vi "Set Pattern.vi"(8 "error in (no error)":errorcluster, 10 "Pattern":string, 11 "Report":refnum<class "Report.lvclass">) -> (0 "error out":errorcluster, 3 "Report out":refnum<class "Report.lvclass">)   [LabVIEW 2011, in "Report.lvclass"]
doc: "This protected method allows the child classes of the report class to set the parent object data.\n\nAAL 9/09"
uses:
  Report.lvclass
  Report.lvclass/Report.ctl
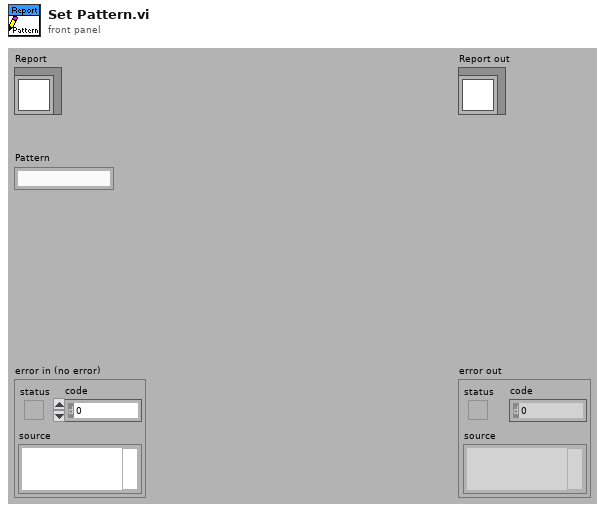
[diagram p1: front panel]
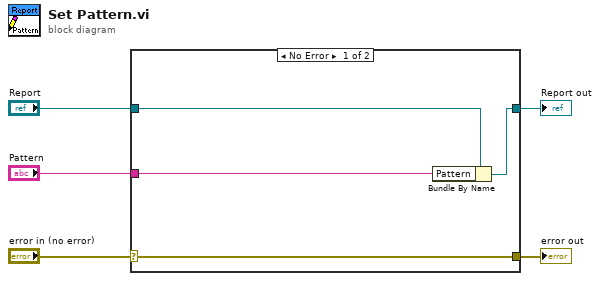
[diagram p0: block diagram]
diagram:
  n1 = case shown="No Error" "error in (no error)" {
    selector: "error in (no error)" -> [w9 w10]
    tunnel: [w9 w10] -> w4
    tunnel: [w7 w11] -> w2
    tunnel: "Report" -> [w8 w11]
    tunnel: "Pattern" -> [w6 _]
    frame No Error {
      n2 = Bundle By Name(cluster=w8, "Pattern"=w6) -> (w7:refnum<class "Report.lvclass">)
    }
    frame Error {
    }
  }
  "error out" <- w4
  "Report out" <- w2
